vi "LogInDialog.vi"(8 "error in (no error)":errorcluster, 10 "Default User":string, 11 "Sequence Context In":refnum<k7>) -> (0 "error out":errorcluster, 1 "Continue?":bool, 2 "UserName":string, 3 "Sequence Context Out":refnum<k7>)   [LabVIEW 2019]
uses:
  <vilib>/addons/TestStand/_TSUtility.llb/TestStand - Start Modal Dialog (Sequence Context).vi
  <vilib>/addons/TestStand/_TSUtility.llb/TestStand - End Modal Dialog (Sequence Context).vi
panel:
  in  "User name:":string(combo)
  in  "Cancel":bool
  in  "OK":bool
  in  "Password:":string
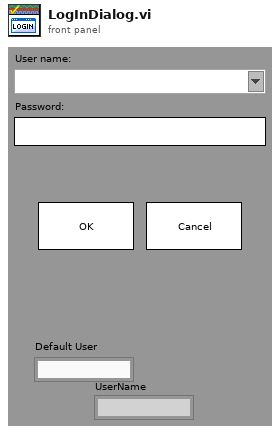
[diagram p1: front panel]
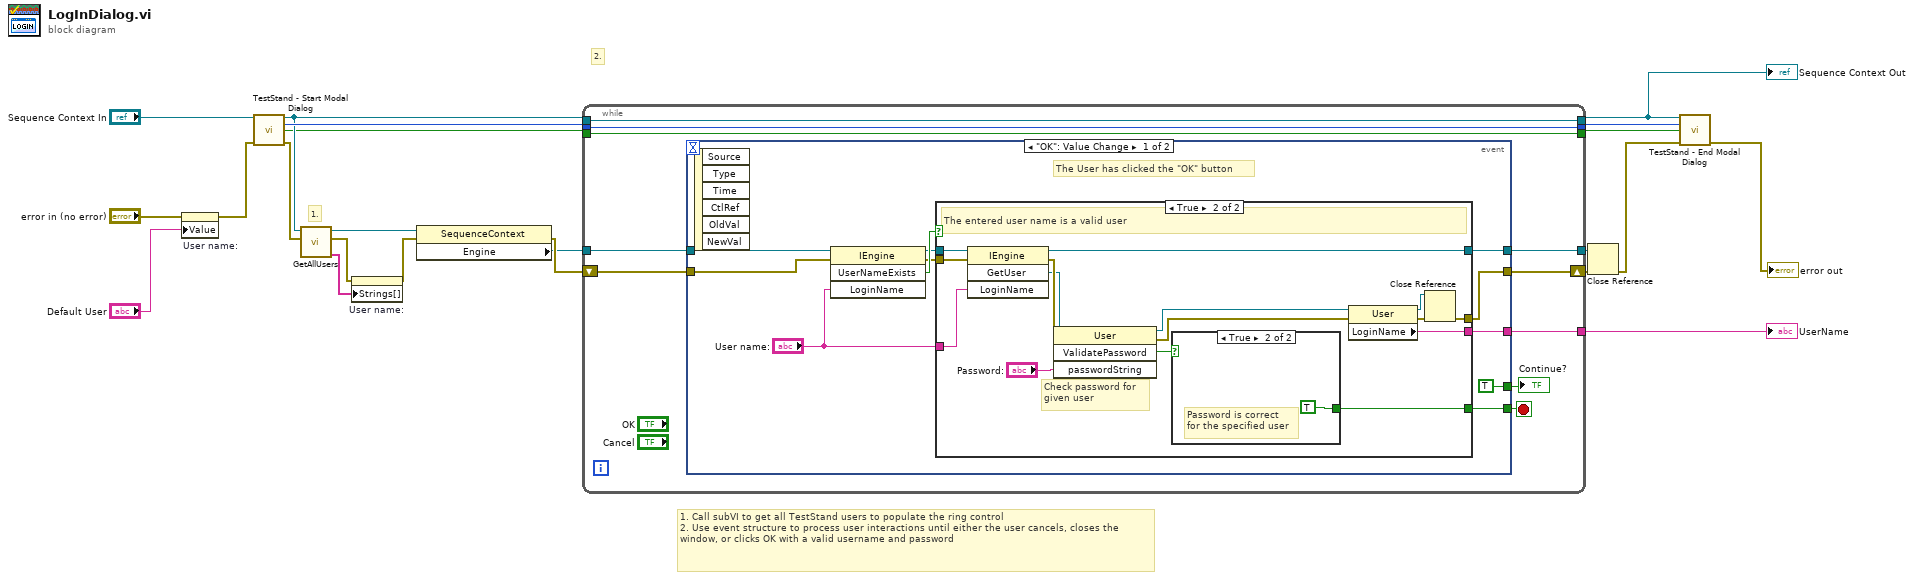
[diagram p0: block diagram]
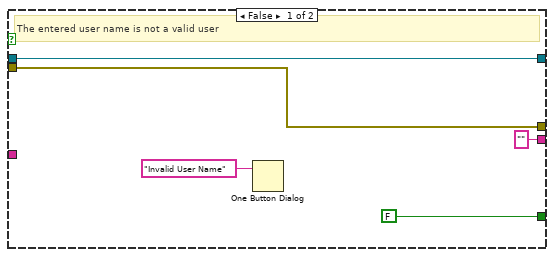
[diagram p2: hidden frame]
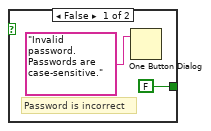
[diagram p3: hidden frame]
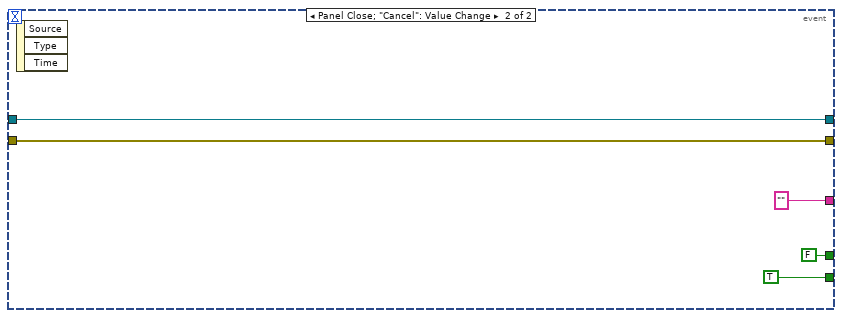
[diagram p4: hidden frame]
diagram:
  # "1. Call subVI to get all TestStand users to populate the ring control\n2. Use event structure to process user interactions until either the user cancels, closes the window, or clicks OK with a valid username and password"
  # "2."
  # "1."
  n1 = property on="User name:" class="CmbBox"(error in="error in (no error)", "Value"="Default User") -> (error out=w4:errorcluster)  [unwired: 1 in, 1 out]
  n2 = call-poly <vilib>:"TestStand - Start Modal Dialog.vi"("Sequence Context In"="Sequence Context In", "error in (no error)"=w4) -> ("Sequence Context Out"=w14:refnum<k7>, "Modal ID"=w15:i32, "VI Originally Open"=w13:bool, "error out"=w22:errorcluster)  [unwired: 9 in, 1 out]
  n3 = call "GetAllUsers.vi"("error in (no error)"=w22, "Sequence Context In"=w14) -> ("Array"=w11:string[], "error out"=w3:errorcluster, "Sequence Context Out"=w21:refnum<k7>)  [unwired: 1 in, 4 out]
  n4 = property on="User name:" class="CmbBox"(error in=w3, "Strings[]"=w11) -> (error out=w2:errorcluster)  [unwired: 1 in, 1 out]
  n5 = property class="SequenceContext"(reference=w21, error in=w2) -> (error out=w19:errorcluster, "Engine"=w10:refnum<k7>)  [unwired: 1 out]
  n6 = while {
    tunnel: w10 -> [w32]
    shift-right: [w29] -> w9
    shift-left: w19 -> [w31]
    tunnel: [w28] -> w18
    tunnel: [w27] -> w16
    tunnel: w15 -> [w27]
    tunnel: w14 -> [w26]
    tunnel: [w26] -> w1
    tunnel: w13 -> [w25]
    tunnel: [w25] -> w12
    tunnel: [w24] -> w8
    stop <- w30 stop-if-true
    n7 = event shown="[0] \"OK\": Value Change" {
      selector: _ -> [_ _]
      dyn-events: _ -> [_ _]
      timeout: _ -> [_ _]
      tunnel: w32 -> [w42 w69]
      tunnel: w31 -> [w34 w70]
      tunnel: [w40 TRUE ("x")] -> w30
      tunnel: [w36 w70] -> w29
      tunnel: [w37 "" ("LoginName")] -> w28
      tunnel: [w38 w69] -> w24
      tunnel: [TRUE ("x") FALSE ("x")] -> w23
      event "OK": Value Change {
        # "The User has clicked the \"OK\" button"
        n8 = event-data() -> ()  [unwired: 7 out]
        n9 = invoke class="IEngine" method="UserNameExists"(reference=w42, error in=w34, "LoginName"="User name:") -> (reference out=w39:refnum<k7>, error out=w41:errorcluster, "UserNameExists"=w43:bool)  [unwired: 1 in, 1 out]
        n10 = case shown="True" w43 {
          tunnel: [FALSE ("x") w62] -> w40
          tunnel: [w46 w51] -> w36
          tunnel: w41 -> [w46 w60]
          tunnel: w39 -> [w45 w61]
          tunnel: [w45 w57] -> w38
          tunnel: "User name:" -> [_ w56]
          tunnel: ["" ("LoginName") w55] -> w37
          frame False {
            # "The entered user name is not a valid user"
            n11 = One Button Dialog(message="Invalid User Name") -> ()  [unwired: 2 out]
          }
          frame True {
            # "Check password for\ngiven user"
            # "The entered user name is a valid user"
            n12 = invoke class="IEngine" method="GetUser"(reference=w61, error in=w60, "LoginName"=w56) -> (reference out=w57:refnum<k7>, error out=w59:errorcluster, "GetUser"=w58:refnum<k7>)  [unwired: 1 in, 1 out]
            n13 = invoke class="User" method="ValidatePassword"(reference=w58, error in=w59, "passwordString"="Password:") -> (reference out=w54:refnum<k7>, error out=w53:errorcluster, "ValidatePassword"=w63:bool)  [unwired: 1 in, 1 out]
            n14 = case shown="True" w63 {
              tunnel: [FALSE ("x") TRUE ("x")] -> w62
              frame False {
                # "Password is incorrect"
                n15 = One Button Dialog(message="Invalid password. Passwords are case-sensitive.") -> ()  [unwired: 2 out]
              }
              frame True {
                # "Password is correct\nfor the specified user"
              }
            }
            n16 = property class="User"(reference=w54, error in=w53) -> (reference out=w50:refnum<k7>, error out=w52:errorcluster, "LoginName"=w55:string)
            n17 = Close Reference(reference=w50, error in (no error)=w52) -> (error out=w51:errorcluster)
          }
        }
      }
      event Panel Close; "Cancel": Value Change {
        n18 = event-data() -> ()  [unwired: 4 out]
      }
    }
    "Continue?" <- w23
  }
  "Sequence Context Out" <- w1
  "UserName" <- w18
  n19 = Close Reference(reference=w8, error in (no error)=w9) -> (error out=w7:errorcluster)
  n20 = call-poly <vilib>:"TestStand - End Modal Dialog.vi"("Sequence Context In"=w1, "Modal ID"=w16, "VI Originally Open"=w12, "error in (no error)"=w7) -> ("error out"=→"error out":errorcluster)  [unwired: 11 in]
